vi "Wait on Notification FGV.vi"(8 "error in":errorcluster, 10 "Get Notifier?":bool, 11 "notifier in":refnum<notifier>) -> (0 "error out":errorcluster, 2 "notification":variant, 3 "notifier out":refnum<notifier>)   [LabVIEW 2020, in "Sequencer Handshake.lvlib"]
doc: "Wait for Notifier FGV.\n\nFUNCTION Gets the notifier reference.\n\nINPUTS\nnotifier in: Reference to be stored in the FGV\nGet Notifier?: TRUE\n\nOUTPUTS\nnotifier out: Reference used by the FGV functions.\nnotification: Empty\n\nFUNCTION (Default) Wait on notification.\n\nInputs\nnotifier in: Ignored.\nGet Notifier?: FALSE\n\nOutputs\nnotifier out: Reference used by the FGV functions.\nnotification: Received variant value.\n\n-----\nJuan Navarro\nLab it Studio"
uses:
  Sequencer Handshake.lvlib
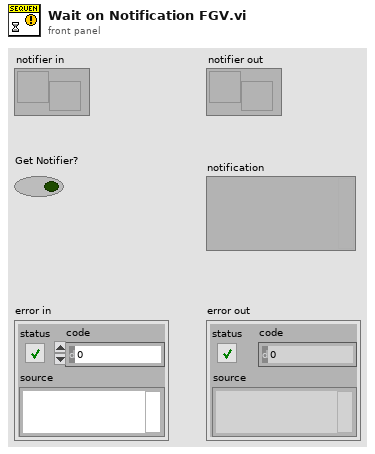
[diagram p1: front panel]
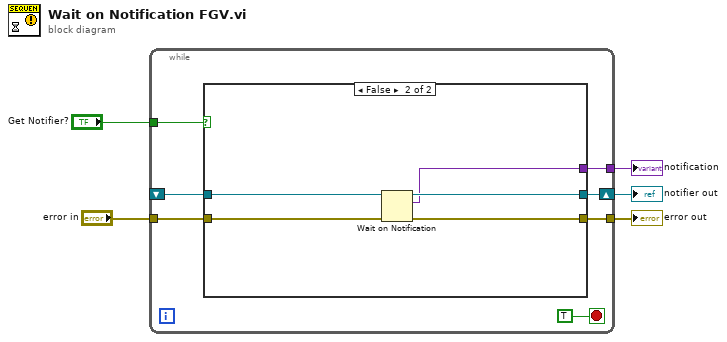
[diagram p0: block diagram]
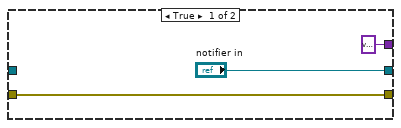
[diagram p2: hidden frame]
diagram:
  n1 = while {
    tunnel: [w12] -> w4
    shift-right: [w11] -> w3
    shift-left: _ -> [w9]
    tunnel: "error in" -> [w10]
    tunnel: "Get Notifier?" -> [w7]
    tunnel: [w6] -> w1
    stop <- TRUE stop-if-true
    n2 = case shown="False" w7 {
      tunnel: w10 -> [w14 w20]
      tunnel: [w14 w19] -> w12
      tunnel: ["notifier in" w17] -> w11
      tunnel: w9 -> [_ w18]
      tunnel: [variant ("element data type") w16] -> w6
      frame True {
      }
      frame False {
        n3 = Wait on Notification(notifier=w18, error in (no error)=w20) -> (notifier out=w17:refnum<notifier>, notification=w16:variant, error out=w19:errorcluster)  [unwired: 2 in, 1 out]
      }
    }
  }
  "error out" <- w4
  "notifier out" <- w3
  "notification" <- w1
